vi "TxPkt - Update Transmit Channels.vi"(4 "Channel Paths":string[](array[string]), 6 "Channel Names":string[](array[string]), 7 "Channle Node Refs":T1[](array[typedef]) format="%.0x", 8 "error in (no error)":errorcluster, 11 "Node Ptr":T1 format="%.0x") -> (0 "error out":errorcluster, 3 "Node Ptr":T1 format="%.0x")   [LabVIEW 2016, in "UDP-Custom-Device System Explorer.lvlib"]
uses:
  UDP-Custom-Device System Explorer.lvlib
  <vilib>/NI Veristand/Custom Device API/Custom Device Item Ref.ctl
  Shared/Types/Shared - Channel Data Type.ctl
  Property Accessors/Tx Packet Accessors.lvlib
  Shared/UDP-Custom-Device Shared.lvlib
  Property Accessors/Shared Packet Accessors.lvlib
  <vilib>/NI VeriStand/Custom Device API/Custom Device API.lvlib
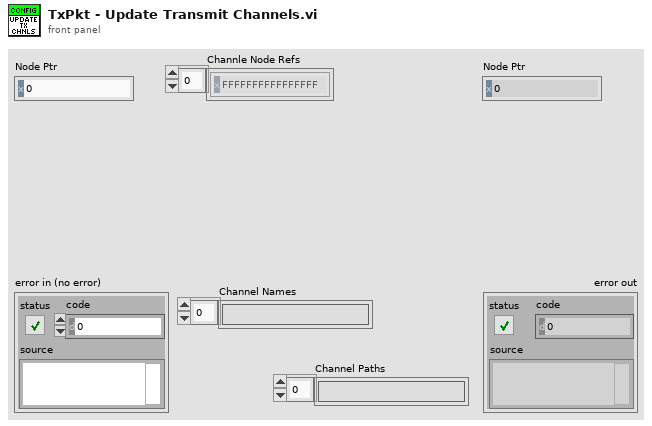
[diagram p1: front panel]
types:
  T1 = typedef "Custom Device API.lvlib/Custom Device Item Ref.ctl" = u64
  T2 = typedef "UDP-Custom-Device Shared.lvlib/Shared - Channel Data Type.ctl" = enum16{"Boolean", "Single", "Double", "I8", "I16", "I32", "I64", "U8", "U16", "U32", "U64"}
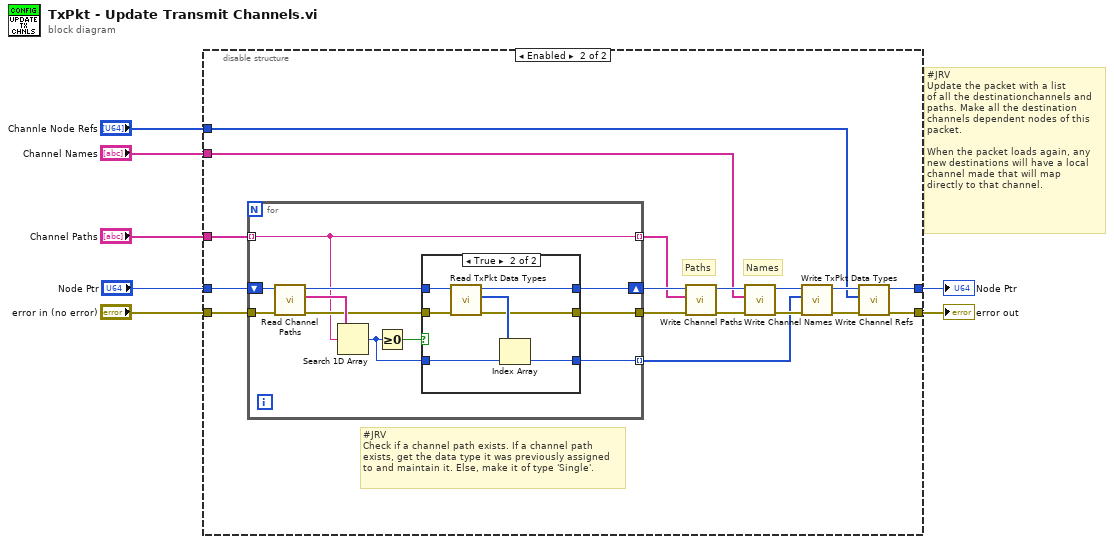
[diagram p0: block diagram]
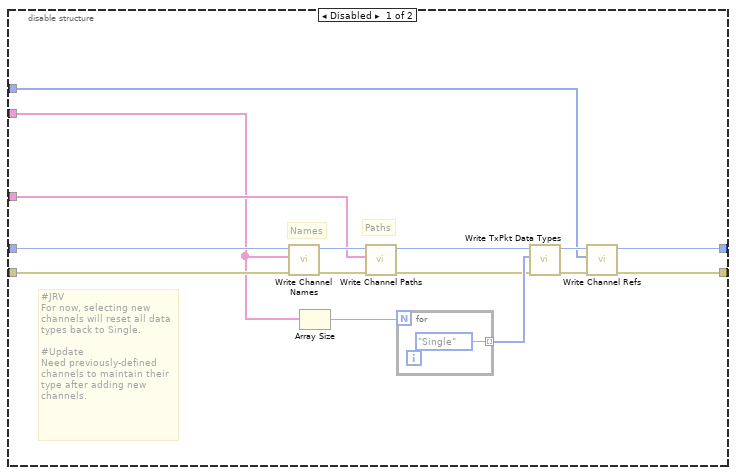
[diagram p2: hidden frame]
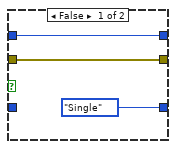
[diagram p3: hidden frame]
diagram:
  # "#JRV\nUpdate the packet with a list\nof all the destinationchannels and\npaths. Make all the destination\nchannels dependent nodes of this\npacket.\n\nWhen the packet loads again, any\nnew destinations will have a local\nchannel made that will map\ndirectly to that channel."
  n1 = disable-structure shown="Enabled" {
    disable-tunnel: [w14 w34] -> w7
    disable-tunnel: "error in (no error)" -> [w13 w39]
    disable-tunnel: "Channle Node Refs" -> [w12 w33]
    disable-tunnel: "Node Ptr" -> [w11 w40]
    disable-tunnel: [w10 w35] -> w3
    disable-tunnel: "Channel Paths" -> [w9 w38]
    disable-tunnel: "Channel Names" -> [w8 w27]
    frame Disabled {
      # "#JRV\nFor now, selecting new\nchannels will reset all data\ntypes back to Single.\n\n#Update\nNeed previously-defined\nchannels to maintain their\ntype after adding new\nchannels."
      # "Paths"
      # "Names"
      n2 = call "Write Channel Names.vi"("error in (no error)"=w13, "Channel Names"=w8, "Node Ptr"=w11) -> ("error out"=w19:errorcluster, "Node Ptr out"=w20:T1)  [unwired: 7 in]
      n3 = Array Size(array=w8) -> (size(s)=w22:i32)
      n4 = call "Write Channel Paths.vi"("error in (no error)"=w19, "Channel Paths"=w9, "Node Ptr"=w20) -> ("error out"=w18:errorcluster, "Node Ptr out"=w17:T1)  [unwired: 7 in]
      n5 = for {
        N: w22 -> [_]
        tunnel: [Shared_-_Channel_Data_Type."Single" ("Data Type")] -> w21 mode=indexing
      }
      n6 = call "Write TxPkt Data Types.vi"("error in (no error)"=w18, "Data Types"=w21, "Node Ptr"=w17) -> ("error out"=w15:errorcluster, "Node Ptr out"=w16:T1)  [unwired: 7 in]
      n7 = call "Write Channel Refs.vi"("error in (no error)"=w15, "Dependent Node Refs"=w12, "Node Ptr"=w16) -> ("error out"=w14:errorcluster, "Node Ptr out"=w10:T1)  [unwired: 7 in]
    }
    frame Enabled {
      # "#JRV\nCheck if a channel path exists. If a channel path\nexists, get the data type it was previously assigned\nto and maintain it. Else, make it of type 'Single'."
      # "Paths"
      # "Names"
      n8 = for {
        tunnel: w39 -> [w50]
        shift-right: [w43] -> w32
        shift-left: w40 -> [w51]
        tunnel: w38 -> [w44] mode=indexing
        tunnel: [w44] -> w30 mode=indexing
        tunnel: [w42] -> w31
        tunnel: [w41] -> w24 mode=indexing
        n9 = call "Read Channel Paths.vi"("error in (no error)"=w50, "Node Ptr"=w51) -> ("error out"=w46:errorcluster, "Channel Paths"=w49:string[], "Node Ptr out"=w45:T1)  [unwired: 7 in]
        n10 = Search 1D Array(1D array=w49, element=w44) -> (index of element=w47:i32)  [unwired: 1 in]
        n11 = Greater Or Equal To 0?(x=w47) -> (x >= 0?=w48:bool)
        n12 = case shown="True" w48 {
          tunnel: w47 -> [_ w58]
          tunnel: w46 -> [w53 w60]
          tunnel: w45 -> [w54 w61]
          tunnel: [w53 w57] -> w42
          tunnel: [w54 w56] -> w43
          tunnel: [Shared_-_Channel_Data_Type."Single" ("Data Type") w55] -> w41
          frame False {
          }
          frame True {
            n13 = call "Read TxPkt Data Types.vi"("error in (no error)"=w60, "Node Ptr"=w61) -> ("error out"=w57:errorcluster, "Data types"=w59:T2[], "Node Ptr out"=w56:T1)  [unwired: 7 in]
            n14 = Index Array(array=w59, index=w58) -> (element=w55:T2)
          }
        }
      }
      n15 = call "Write Channel Paths.vi"("error in (no error)"=w31, "Channel Paths"=w30, "Node Ptr"=w32) -> ("error out"=w28:errorcluster, "Node Ptr out"=w29:T1)  [unwired: 7 in]
      n16 = call "Write Channel Names.vi"("error in (no error)"=w28, "Channel Names"=w27, "Node Ptr"=w29) -> ("error out"=w25:errorcluster, "Node Ptr out"=w26:T1)  [unwired: 7 in]
      n17 = call "Write TxPkt Data Types.vi"("error in (no error)"=w25, "Data Types"=w24, "Node Ptr"=w26) -> ("error out"=w36:errorcluster, "Node Ptr out"=w37:T1)  [unwired: 7 in]
      n18 = call "Write Channel Refs.vi"("error in (no error)"=w36, "Dependent Node Refs"=w33, "Node Ptr"=w37) -> ("error out"=w34:errorcluster, "Node Ptr out"=w35:T1)  [unwired: 7 in]
    }
  }
  "error out" <- w7
  "Node Ptr" <- w3
